vi "exit.vi"(8 "error in (no error)":errorcluster, 11 "Hardware in":refnum<class "Hardware.lvclass">) -> (0 "error out":errorcluster, 3 "Hardware out":refnum<class "Hardware.lvclass">)   [LabVIEW 2016, in "Hardware.lvlib" / "Hardware.lvclass"]
uses:
  Hardware.lvclass
  Hardware.lvclass/Hardware.ctl
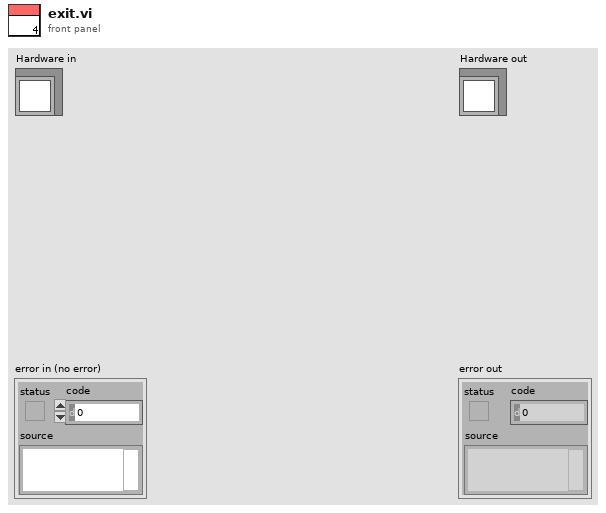
[diagram p1: front panel]
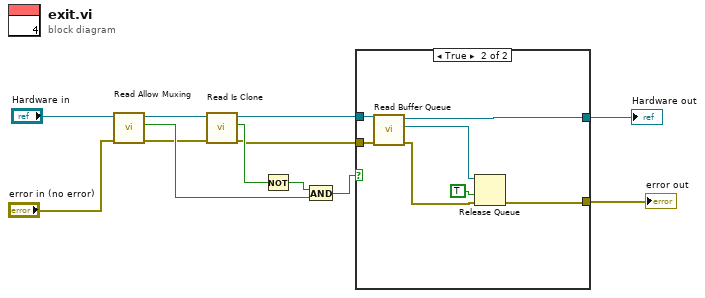
[diagram p0: block diagram]
diagram:
  n1 = call "Read Allow Muxing.vi"("error in (no error)"="error in (no error)", "Hardware in"="Hardware in") -> ("error out"=w3:errorcluster, "Allow Muxing"=w9:bool, "Hardware out"=w8:refnum<class "Hardware.lvclass">)  [unwired: 7 in]
  n2 = call "Read Is Clone.vi"("error in (no error)"=w3, "Hardware in"=w8) -> ("error out"=w2:errorcluster, "Is Clone?"=w11:bool, "Hardware out"=w7:refnum<class "Hardware.lvclass">)  [unwired: 7 in]
  n3 = Not(x=w11) -> (.not. x?=w10:bool)
  n4 = And(x=w10, y=w9) -> (x .and. y?=w4:bool)
  n5 = case shown="True" w4 {
    tunnel: w7 -> [w14 w21]
    tunnel: [w13 w17] -> w6
    tunnel: [w14 w16] -> w5
    tunnel: w2 -> [w13 w15]
    frame False {
    }
    frame True {
      n6 = call "Read Buffer Queue.vi"("error in (no error)"=w15, "Hardware in"=w21) -> ("error out"=w18:errorcluster, "Buffer Queue"=w20:refnum<queue>, "Hardware out"=w16:refnum<class "Hardware.lvclass">)  [unwired: 7 in]
      n7 = Release Queue(queue=w20, force destroy? (F)=TRUE, error in (no error)=w18) -> (error out=w17:errorcluster)  [unwired: 2 out]
    }
  }
  "error out" <- w6
  "Hardware out" <- w5
